vi "메뉴도구바(SubVI).vi"(8 "에러 입력(에러 없음)":errorcluster, 10 "메뉴바/도구바":bool, 11 "VI 입력":refnum<vi>) -> (0 "에러 출력":errorcluster, 3 "VI 출력":refnum<vi>)   [LabVIEW 2014]
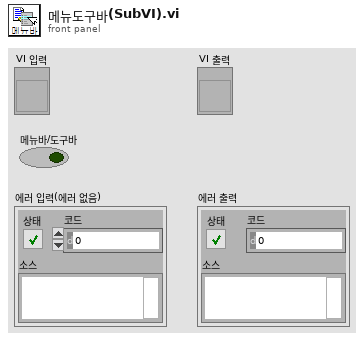
[diagram p1: front panel]
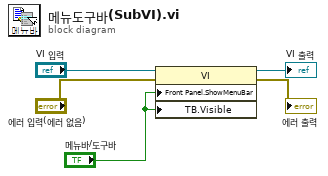
[diagram p0: block diagram]
diagram:
  n1 = property class="VI"(reference="VI 입력", error in="에러 입력(에러 없음)", "Front Panel.ShowMenuBar"="메뉴바/도구바", "TB.Visible"="메뉴바/도구바") -> (reference out=→"VI 출력":refnum<vi>, error out=→"에러 출력":errorcluster)
